vi "Filtri segnali PB.vi"(9 "sampling freq: fs":dbl=1.0 format="%0.2f", 10 "Array":T1(array[cluster]) {"low cutoff freq: fl" format="%0.4f"}, 11 "data in":waveform(dbl)[](array[waveform])) -> (3 "filtered":waveform(dbl)[](array[waveform]))   [LabVIEW 2019]
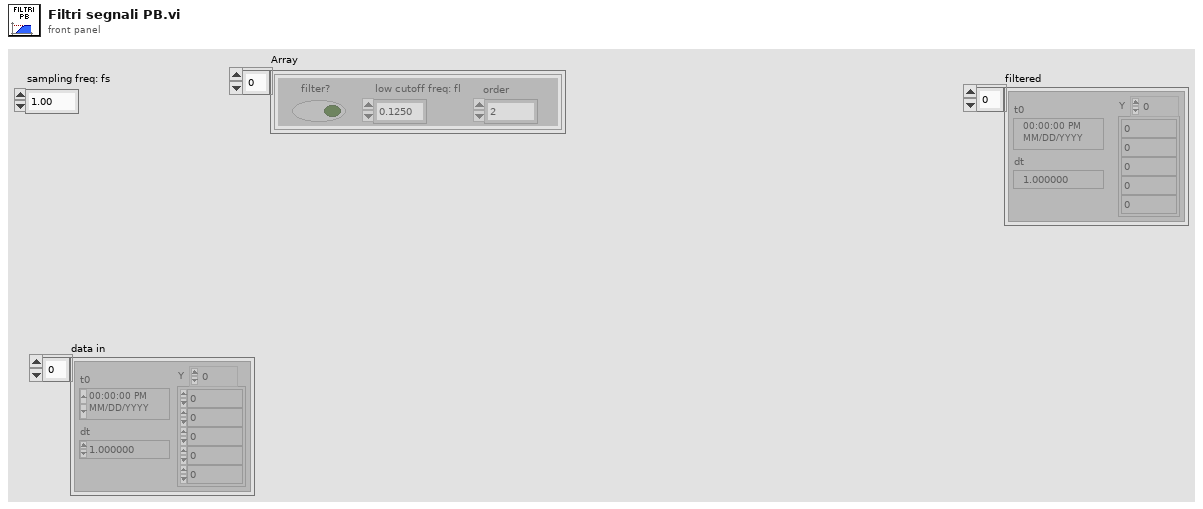
[diagram p1: front panel]
types:
  T1 = cluster{"filter?":bool, "low cutoff freq: fl":dbl, "order":i32}[]
  T2 = cluster{"filter?":bool, "low cutoff freq: fl":dbl, "order":i32}
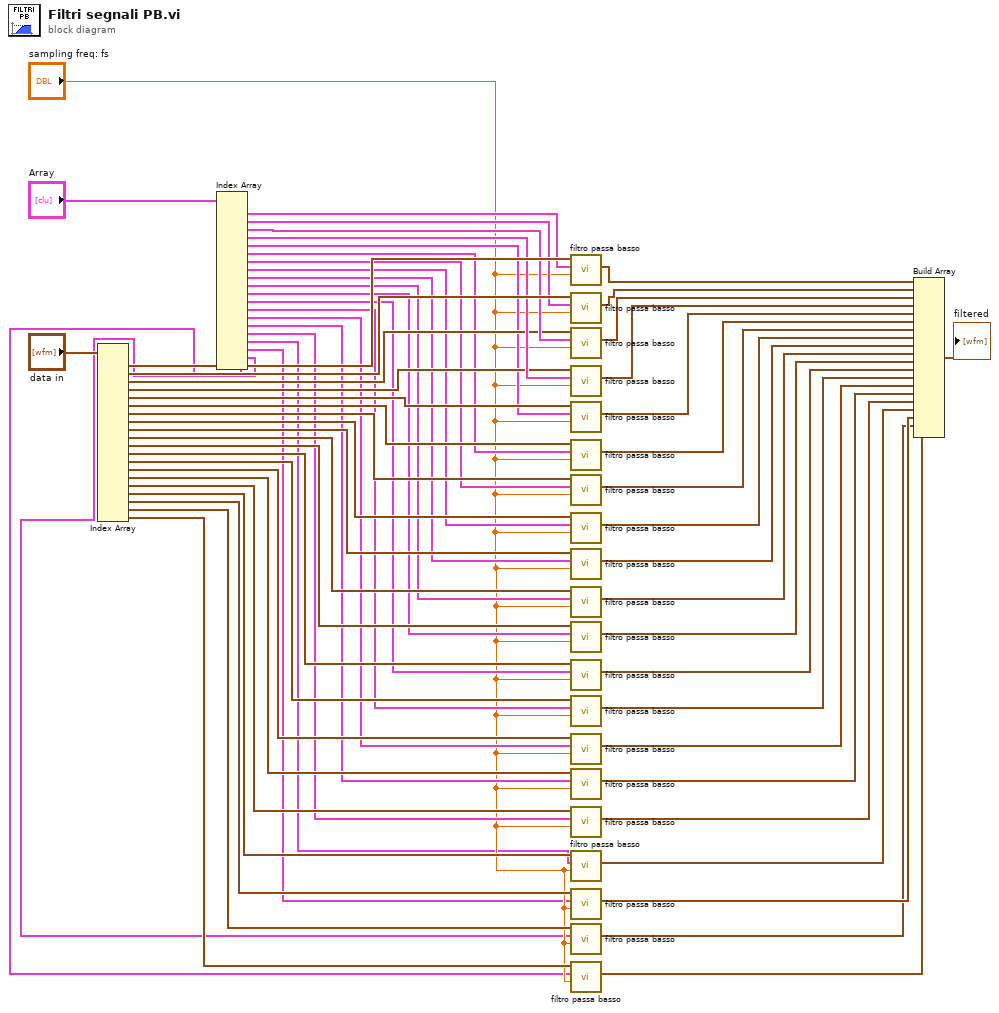
[diagram p0: block diagram]
diagram:
  n1 = Index Array(array="data in") -> (element #1=w64:waveform(dbl), element #2=w60:waveform(dbl), element #3=w56:waveform(dbl), element #4=w55:waveform(dbl), element #5=w54:waveform(dbl), element #6=w52:waveform(dbl), element #7=w50:waveform(dbl), element #8=w48:waveform(dbl), element #9=w46:waveform(dbl), element #10=w45:waveform(dbl), element #11=w44:waveform(dbl), element #12=w43:waveform(dbl), element #13=w42:waveform(dbl), element #14=w41:waveform(dbl), element #15=w40:waveform(dbl), element #16=w39:waveform(dbl), element #17=w13:waveform(dbl), element #18=w12:waveform(dbl), element #19=w11:waveform(dbl), element #20=w10:waveform(dbl))  [unwired: 20 in]
  n2 = Index Array(array="Array") -> (element #1=w61:T2, element #2=w59:T2, element #3=w58:T2, element #4=w57:T2, element #5=w53:T2, element #6=w51:T2, element #7=w49:T2, element #8=w47:T2, element #9=w38:T2, element #10=w37:T2, element #11=w36:T2, element #12=w35:T2, element #13=w34:T2, element #14=w33:T2, element #15=w32:T2, element #16=w31:T2, element #17=w8:T2, element #18=w7:T2, element #19=w6:T2, element #20=w5:T2)  [unwired: 20 in]
  n3 = call "filtro passa basso.vi"("sampling freq: fs"="sampling freq: fs", "Cluster"=w61, "Waveform"=w64) -> ("Waveform 2"=w30:waveform(dbl))  [unwired: 8 in]
  n4 = call "filtro passa basso.vi"("sampling freq: fs"="sampling freq: fs", "Cluster"=w59, "Waveform"=w60) -> ("Waveform 2"=w29:waveform(dbl))  [unwired: 8 in]
  n5 = call "filtro passa basso.vi"("sampling freq: fs"="sampling freq: fs", "Cluster"=w58, "Waveform"=w56) -> ("Waveform 2"=w28:waveform(dbl))  [unwired: 8 in]
  n6 = call "filtro passa basso.vi"("sampling freq: fs"="sampling freq: fs", "Cluster"=w57, "Waveform"=w55) -> ("Waveform 2"=w27:waveform(dbl))  [unwired: 8 in]
  n7 = call "filtro passa basso.vi"("sampling freq: fs"="sampling freq: fs", "Cluster"=w53, "Waveform"=w54) -> ("Waveform 2"=w26:waveform(dbl))  [unwired: 8 in]
  n8 = call "filtro passa basso.vi"("sampling freq: fs"="sampling freq: fs", "Cluster"=w51, "Waveform"=w52) -> ("Waveform 2"=w25:waveform(dbl))  [unwired: 8 in]
  n9 = call "filtro passa basso.vi"("sampling freq: fs"="sampling freq: fs", "Cluster"=w49, "Waveform"=w50) -> ("Waveform 2"=w24:waveform(dbl))  [unwired: 8 in]
  n10 = call "filtro passa basso.vi"("sampling freq: fs"="sampling freq: fs", "Cluster"=w47, "Waveform"=w48) -> ("Waveform 2"=w23:waveform(dbl))  [unwired: 8 in]
  n11 = call "filtro passa basso.vi"("sampling freq: fs"="sampling freq: fs", "Cluster"=w38, "Waveform"=w46) -> ("Waveform 2"=w22:waveform(dbl))  [unwired: 8 in]
  n12 = call "filtro passa basso.vi"("sampling freq: fs"="sampling freq: fs", "Cluster"=w37, "Waveform"=w45) -> ("Waveform 2"=w21:waveform(dbl))  [unwired: 8 in]
  n13 = call "filtro passa basso.vi"("sampling freq: fs"="sampling freq: fs", "Cluster"=w36, "Waveform"=w44) -> ("Waveform 2"=w20:waveform(dbl))  [unwired: 8 in]
  n14 = call "filtro passa basso.vi"("sampling freq: fs"="sampling freq: fs", "Cluster"=w35, "Waveform"=w43) -> ("Waveform 2"=w19:waveform(dbl))  [unwired: 8 in]
  n15 = call "filtro passa basso.vi"("sampling freq: fs"="sampling freq: fs", "Cluster"=w34, "Waveform"=w42) -> ("Waveform 2"=w18:waveform(dbl))  [unwired: 8 in]
  n16 = call "filtro passa basso.vi"("sampling freq: fs"="sampling freq: fs", "Cluster"=w33, "Waveform"=w41) -> ("Waveform 2"=w17:waveform(dbl))  [unwired: 8 in]
  n17 = call "filtro passa basso.vi"("sampling freq: fs"="sampling freq: fs", "Cluster"=w32, "Waveform"=w40) -> ("Waveform 2"=w16:waveform(dbl))  [unwired: 8 in]
  n18 = call "filtro passa basso.vi"("sampling freq: fs"="sampling freq: fs", "Cluster"=w31, "Waveform"=w39) -> ("Waveform 2"=w15:waveform(dbl))  [unwired: 8 in]
  n19 = call "filtro passa basso.vi"("sampling freq: fs"="sampling freq: fs", "Cluster"=w8, "Waveform"=w13) -> ("Waveform 2"=w4:waveform(dbl))  [unwired: 8 in]
  n20 = call "filtro passa basso.vi"("sampling freq: fs"="sampling freq: fs", "Cluster"=w7, "Waveform"=w12) -> ("Waveform 2"=w3:waveform(dbl))  [unwired: 8 in]
  n21 = call "filtro passa basso.vi"("sampling freq: fs"="sampling freq: fs", "Cluster"=w6, "Waveform"=w11) -> ("Waveform 2"=w2:waveform(dbl))  [unwired: 8 in]
  n22 = call "filtro passa basso.vi"("sampling freq: fs"="sampling freq: fs", "Cluster"=w5, "Waveform"=w10) -> ("Waveform 2"=w1:waveform(dbl))  [unwired: 8 in]
  n23 = Build Array(w30, w29, w28, w27, w26, w25, w24, w23, w22, w21, w20, w19, w18, w17, w16, w15, w4, w3, w2, w1) -> (→"filtered":waveform(dbl)[])
